vi "PH_Cont-601k_PowerUnit.set i Attr and open Services.vi"(0 "i ref in":refnum<vi>, 5 "error in":errorcluster) -> (14 "i ref out":refnum<vi>, 16 "i Attribhutes":T1={"Service ID Last Shot"=-1}, 19 "error out":errorcluster)   [LabVIEW 2014, in "PH_Cont-601k_PowerUnit.lvlib"]
doc: "In this VI the related instances which are not set in Read DB are set and written to own attributes."
uses:
  PH_Cont-601k_PowerUnit.lvlib
  PH_Cont-601k_PowerUnit.i attribute.ctl
  PH_Basics/PH_PP_Common/PH_PP_Common.Trigger Tags.ctl
  PH_Basics/PH_PP_Common/PH_PP_Common.lvlib
  CSlibraries-extern/DimLVEvent/LVDimInterface/LVDimInterface.lvlib
  PH_Basics/PH_PowerUnit_BaseClass/PH_PowerUnit_BaseClass.lvlib
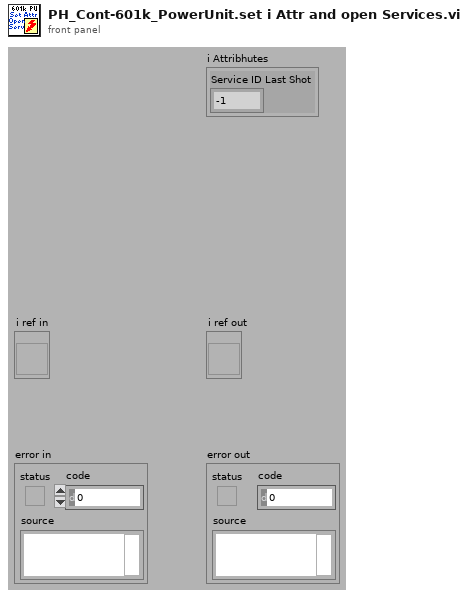
[diagram p1: front panel]
types:
  T1 = typedef "PH_Cont-601k_PowerUnit.lvlib/PH_Cont-601k_PowerUnit.i attribute.ctl" = cluster{"Service ID Last Shot":i32}
  T2 = typedef "PH_PP_Common.lvlib/PH_PP_Common.Trigger Tags.ctl" = enum16{"triggered", "fired", "Status", "Last Shot"}
  T3 = typedef "PH_PowerUnit_BaseClass.lvlib/PH_PowerUnit_BaseClass.i attribute.ctl" = cluster{"Constructor finished":bool, "PU":cluster{"In use":bool, "Service ID in use":i32, "GUI Ref":refnum<vi>}, "Enabling":cluster{"State":T4, "GUI Ref":refnum<vi>}, "Timing":cluster{"Last Shot":dbl, "Time between Shots [Sec]":dbl, "Waiting Time over?":bool, "Service ID Waiting Time":i32, "GUI Ref":refnum<vi>, "Instance":cluster{"Status":T5, "linked?":bool, "GUI Ref":refnum<vi>}}, "Sequencer":cluster{"SM State":string, "GUI Ref":refnum<vi>, "linked":bool}, "Subscribed Trendmssgs":cluster{"Tagname":string, "Status":T5, "linked?":bool, "Shot Condition":T5, "GUI Ref":refnum<vi>}[], "PP PU":T6, "Default Voltage (V)":dbl, "GUI Refs":T7, "PSDB data":cluster{"Shot Voltage [V]":dbl, "State TO SM":T8, "Write 2 early":bool}, "State TO SM":T8}
  T4 = typedef "PH_SystemInformation.lvlib/PH_SystemInformationEnabling State.ctl" = i32
  T5 = typedef "PH_StatusHandler.lvlib/PH_StatusHandler.Status.ctl" = i16
  T6 = typedef "PH_PP_Common.lvlib/PH_PP_Common.PUs.ctl" = enum16{"no Info", "PA-19mm-1", "PA-19mm-2", "PA-45mm-PILC", "PA-45mm-MAIN", "MA-PU-1", "MA-PU-2", "MA-PU-3", "MA-PU-4", "MA-PU-5", "MA-PU-6", "MA-FR", "MA-PILC", "PA-45mm-DP"}
  T7 = typedef "PH_PowerUnit_BaseClass.lvlib/PH_PowerUnit_BaseClass.GUI Refs.ctl" = cluster{"Delete Inst":refnum<vi>, "State TO SM":refnum<vi>, "State SM":refnum<vi>, "Fire":refnum<vi>}
  T8 = typedef "PH_PowerUnit_BaseClass.lvlib/PH_PowerUnit_BaseClass.SM States.ctl" = enum16{".", "Stand by", "Switch PU on", "Configure", "Set Default Voltage", "Set STANDBY", "Set READY", "Wait for Shot Cmd", "Open Dump Rods", "Open Ross Relais", "Close Ross Relais", "Switch PSU on", "Switch PSU off", "Charge", "Switch GD Channel on", "Close Dump Rods", "Rods-TO", "RR-TO", "PSU-TO", "Trigger-TO"}
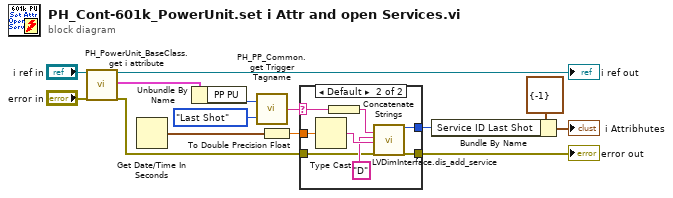
[diagram p0: block diagram]
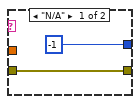
[diagram p2: hidden frame]
diagram:
  n1 = call "PH_PowerUnit_BaseClass.get i attribute.vi"("i ref in"="i ref in", "error in (no error)"="error in") -> ("i ref out"=→"i ref out":refnum<vi>, "i attribute"=w2:T3, "error out"=w5:errorcluster)  [unwired: 15 in]
  n2 = Get Date/Time In Seconds() -> (seconds since 1Jan1904=w13:timestamp)
  n3 = Unbundle By Name(w2) -> ("PP PU"=w1:T6)
  n4 = call "PH_PP_Common.get Trigger Tagname.vi"("Trigger Tag"=PH_PP_Common.Trigger_Tags."Last Shot", "PU"=w1) -> ("Trigger Tagname"=w9:string)
  n5 = To Double Precision Float(number=w13) -> (double precision float=w10:dbl)
  n6 = case shown="Default" w9 {
    selector: w9 -> [_ w19]
    tunnel: [-1 ("my_serviceID") w18] -> w8
    tunnel: [w16 w20] -> w7
    tunnel: w5 -> [w16 w21]
    tunnel: w10 -> [_ w17]
    frame "N/A" {
    }
    frame Default {
      n7 = Type Cast(x=w17) -> (*(type *) &x=w24:string)  [unwired: 1 in]
      n8 = Concatenate Strings(w19) -> (w22:string)
      n9 = call "LVDimInterface.dis_add_service.vi"("serviceName"=w22, "typeDescriptor"="D", "data"=w24, "error in (no error)"=w21) -> ("my_serviceID"=w18:i32, "error out"=w20:errorcluster)  [unwired: 14 in]
    }
  }
  "error out" <- w7
  n10 = Bundle By Name(cluster=T1 {"Service ID Last Shot"=-1} ("i attribute"), "Service ID Last Shot"=w8) -> (→"i Attribhutes":T1)
